vi "Write Position Props.vi"(8 "error in (no error)":errorcluster, 10 "Position Props":T1, 11 "Ctl Refnum in":refnum<vi>) -> (0 "error out":errorcluster, 3 "Ctl Refnum":refnum<vi>)   [LabVIEW 2020, in "VolatusGUIEditorCore.lvlib"]
uses:
  VolatusGUIEditorCore.lvlib
  Position Props.ctl
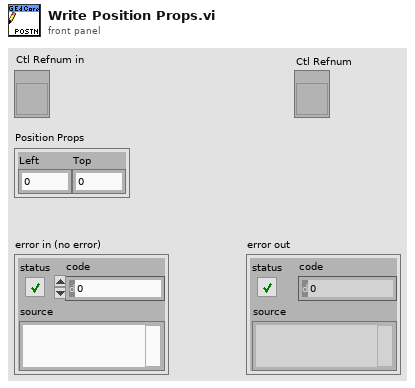
[diagram p1: front panel]
types:
  T1 = typedef "VolatusGUIEditorCore.lvlib/Position Props.ctl" = cluster{"Left":i32, "Top":i32}
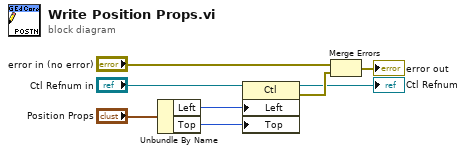
[diagram p0: block diagram]
diagram:
  n1 = Unbundle By Name("Position Props") -> ("Left"=w5:i32, "Top"=w6:i32)
  n2 = property class="Ctl"(reference="Ctl Refnum in", "Left"=w5, "Top"=w6) -> (reference out=→"Ctl Refnum":refnum<vi>, error out=w3:errorcluster)  [unwired: 1 in]
  n3 = Merge Errors("error in (no error)", w3) -> (→"error out":errorcluster)
